vi "Hex to Flattened String.vi"(1 "Hex":string) -> (0 "Flattened String":string)   [LabVIEW 2016, in "Configit.lvlib"]
uses:
  Configit.lvlib
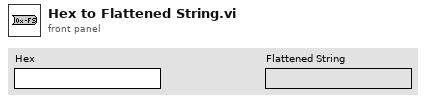
[diagram p1: front panel]
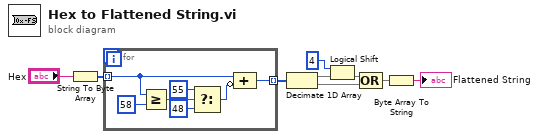
[diagram p0: block diagram]
diagram:
  n1 = String To Byte Array(string="Hex") -> (unsigned byte array=w2:u8[])
  n2 = for {
    tunnel: w2 -> [w14] mode=indexing
    tunnel: [w16] -> w1 mode=indexing
    n3 = Greater Or Equal?(x=w14, y=u8 58) -> (x >= y?=w12:bool)
    n4 = Select(t=u8 55 ("value"), s=w12, f=u8 48 ("value")) -> (s? t:f=w15:u8)
    n5 = Compound Arithmetic op=ADD(w14, invert w15) -> (w16:u8)
  }
  n6 = Decimate 1D Array(w1) -> (w7:u8[], w6:u8[])
  n7 = Logical Shift(y=i8 4, x=w7) -> (x << y=w8:u8[])
  n8 = Compound Arithmetic op=OR(w8, w6) -> (w4:u8[])
  n9 = Byte Array To String(unsigned byte array=w4) -> (string=→"Flattened String":string)
